vi "ChangeAmpWFG.vi"(0 "object in":refnum<class "AD2_SDK.lvclass">, 2 "AmplitudeCh1&2":T1, 5 "error in (no error)":errorcluster) -> (14 "object out":refnum<class "AD2_SDK.lvclass">, 19 "error out":errorcluster)   [LabVIEW 2021, in "AD2_SDK.lvclass"]
uses:
  AD2_SDK.lvclass
  AD2_SDK.lvclass/AD2_SDK.ctl
  AD2_WFG_SDK_class/AD2_WFG_SDK.lvclass
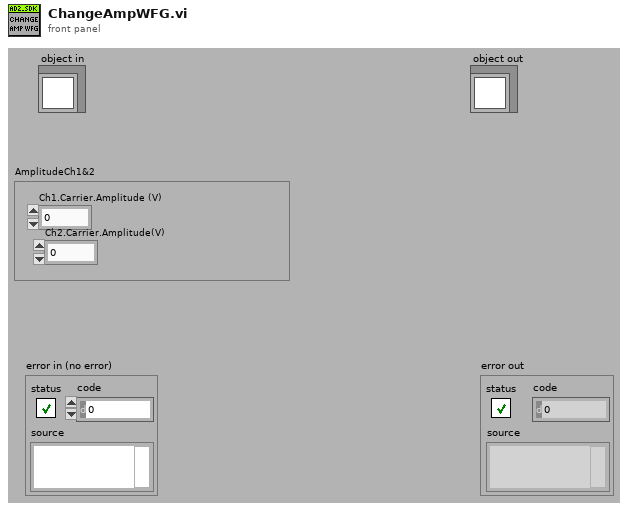
[diagram p1: front panel]
types:
  T1 = cluster{"Ch1.Carrier.Amplitude (V)":dbl, "Ch2.Carrier.Amplitude(V)":dbl}
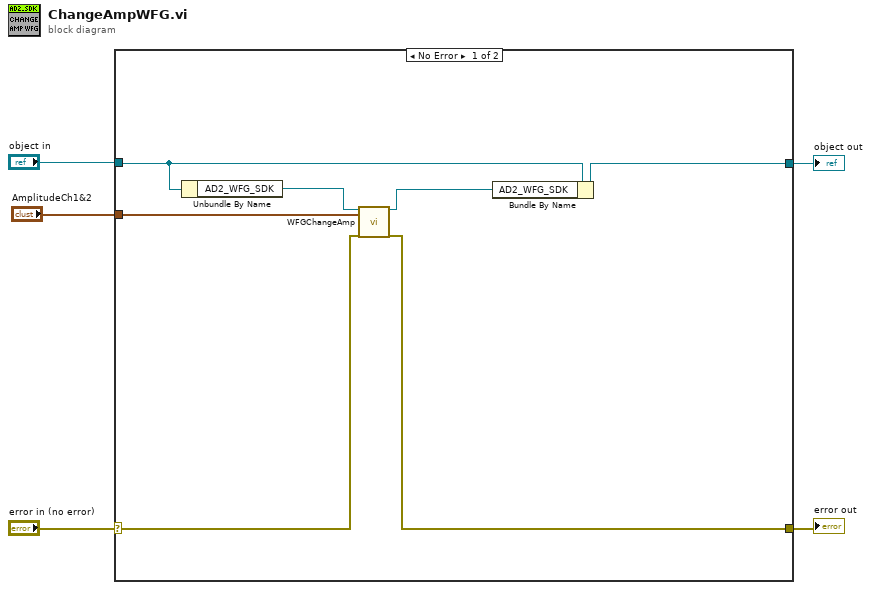
[diagram p0: block diagram]
diagram:
  n1 = case shown="No Error" "error in (no error)" {
    selector: "error in (no error)" -> [w8 w14]
    tunnel: [w7 w14] -> w4
    tunnel: [w11 w13] -> w2
    tunnel: "object in" -> [w12 w13]
    tunnel: "AmplitudeCh1&2" -> [w6 _]
    frame No Error {
      n2 = Unbundle By Name(w12) -> ("AD2_WFG_SDK"=w10:refnum<class "AD2_WFG_SDK.lvclass">)
      n3 = call-dynamic "WFGChangeAmp.vi"("object in"=w10, "AmplitudeCh1&2"=w6, "error in (no error)"=w8) -> ("object out"=w9:refnum<class "AD2_WFG_SDK.lvclass">, "error out"=w7:errorcluster)  [unwired: 15 in]
      n4 = Bundle By Name(cluster=w12, "AD2_WFG_SDK"=w9) -> (w11:refnum<class "AD2_SDK.lvclass">)
    }
    frame Error {
    }
  }
  "error out" <- w4
  "object out" <- w2
